vi "Lidar V3 RT Main.vi"() -> ()   [LabVIEW 2013]
uses:
  <vilib>/Platform/TimedLoop/XDataNode/timing_clust.ctl
  <vilib>/Platform/TimedLoop/XDataNode/nitl_modes.ctl
  <vilib>/Platform/TimedLoop/XDataNode/wakeup.ctl
  <vilib>/FPGAPlugInAG/PXIe-7962R/niLvFpga_Open_PXIe-7962R.vi
  <vilib>/rvi/interface/common/dynamic/niFpgaDynamicAddResources.vi
  <vilib>/FPGAPlugInAG/Dynamic/niLvFpga_Abort_Dynamic.vi
  <vilib>/FPGAPlugInAG/Dynamic/niLvFpga_Reset_Dynamic.vi
  <vilib>/FPGAPlugInAG/Dynamic/niLvFpga_Run_Dynamic.vi
  <vilib>/rvi/interface/common/niFpgaWaitOnOcc.vi
  <vilib>/Utility/error.llb/Error Cluster From Error Code.vi
  <vilib>/rvi/errors/niLvFpgaAdjustHostInterfaceError.vi
  <vilib>/FPGAPlugInAG/Dynamic/niLvFpga_Close_Dynamic.vi
  <vilib>/rvi/interface/nirviOpenFPGA/nirviOpenFPGA.xnode
  FPGA Bitfiles/LIDAR Module 5782 V3.2.lvbitx
  <vilib>/rvi/interface/nirviMethod/nirviMethod.xnode
  <vilib>/Platform/TimedLoop/XDataNode/XDataNode.xnode
  <vilib>/rvi/interface/nirviReadWriteControl/nirviReadWriteControl.xnode
  <vilib>/rvi/interface/nirviCloseFPGA/nirviCloseFPGA.xnode
  <vilib>/FPGAPlugInAG/Dynamic/niLvFpga_ReadFifo_Dynamic.vi
  <vilib>/rvi/errors/niLvFpgaMergeErrorWithErrorCode.vi
  <vilib>/ptbypt/NI_PtbyPt.lvlib
  NiFpgaLv.dll
  <vilib>/rvi/interface/Simulation/niFpgaSimulationCallBeginRW.vi
  <vilib>/Platform/TimedLoop/XDataNode/XDNodeRunTimeDep.lvlib
  <vilib>/FPGAPlugInAG/Dynamic/niLvFpga_StopFifo_Dynamic.vi
  <vilib>/FPGAPlugInAG/Dynamic/niLvFpga_ConfigureFifo_Dynamic.vi
  <vilib>/FPGAPlugInAG/Dynamic/niLvFpga_AcquireReadRegionFifo_Dynamic.vi
panel:
  out "frames counter":u32
  in  "# of Frames":u32=100
  in  "Frames Stream":bool
  in  "Frames Period":i64=100
  out "Actual Depth":u32=400384
  out "Raw Data Timeouts":u16
  in  "StreamToRawFile":bool
  in  "SingleFrame":bool
  in  "SamplingEnable":bool=TRUE
  out "Elements":i32=89152
  out "DiskWritesCounter":dbl=375.0
  out "error out 2":errorcluster
  in  "Write To File":bool
  in  "file path (use dialog)":path=path "C:/Users/LIDAR/Desktop/Scans/InterScan4.dat"
  out "error out 3":errorcluster
  out "Elements Remaining":u32
  in  "MaxStartSample":u8
  out "Intensity Map":u32[][](graph)=[[129791, 129680, 130020, 129704, 129932, 129336, 129397, 129600, 129645, 130103, 129648, 130030, 129625, 129970, 129708, 129573], [129593, 129680, 130141, 129910, 129596, 129500, 129521, 129569, 129949, 129774, 129846, 129832, 129809, 129824, 130165, 129650], [129735, 129752, 129871, 130235, 129687, 129440, 129980, 129667, 129799, 129541, 129983, 129757, 129478, 129736, 129657, 129715], [129751, 129583, 129677, 129965, 129579, 129714, 129407, 129739, 129751, 129654, 129836, 129799, 129748, 129751, 130116, 129495], [129571, 129639, 130270, 129388, 129740, 129773, 129237, 129955, 129670, 129830, 130261, 129436, 130070, 129727, 129314, 129829], [129652, 129843, 130032, 129955, 129968, 129379, 129685, 130041, 129814, 129499, 129706, 129869, 129869, 129962, 129707, 129878], [129807, 129828, 130008, 129984, 129406, 129957, 129543, 130066, 129909, 130276, 129623, 129692, 130095, 130106, 129557, 129714], [129986, 130220, 129551, 130069, 129832, 129932, 129900, 129936, 129877, 129862, 129771, 129582, 129720, 129949, 129916, 129711], [129633, 129877, 130052, 130093, 130030, 129994, 129636, 129905, 129789, 130086, 129907, 129523, 129744, 129981, 129449, 129771], [129913, 129683, 129520, 129782, 129841, 129742, 129616, 129954, 129366, 129733, 129625, 129664, 129876, 129869, 129544, 129710], [129901, 129619, 129661, 130086, 129825, 129761, 129804, 129725, 129375, 130051, 129757, 129787, 129999, 129670, 130011, 130055], [129946, 129776, 130199, 129713, 129738, 129633, 129897, 129662, 129661, 129515, 129708, 129511, 130068, 129836, 129857, 129680], [129649, 129866, 129818, 130111, 129942, 129748, 129540, 129872, 130033, 129595, 129906, 129804, 129753, 129581, 130001, 129824], [129533, 129412, 129678, 129388, 130078, 129617, 129776, 130004, 129502, 129913, 129651, 129903, 129629, 130071, 130057, 129771], [129683, 129809, 130073, 130027, 129777, 129962, 129746, 129781, 129655, 129602, 129804, 129795, 129831, 130156, 129740, 130062], [130093, 129615, 129781, 129920, 129948, 129767, 129590, 129269, 129763, 129611, 129844, 129676, 129702, 130070, 129930, 129907], [129766, 130025, 130030, 129536, 130034, 130049, 129643, 129787, 129735, 129792, 129751, 129963, 129966, 129726, 129589, 129781], [129637, 129588, 129765, 129794, 129683, 129663, 129966, 129384, 129794, 129709, 129656, 129867, 129751, 129686, 129595, 129758], [129833, 129773, 129371, 130164, 129799, 129859, 129589, 129792, 129484, 129830, 130126, 130134, 129838, 129988, 129646, 129826], [129864, 129971, 129896, 129600, 129709, 129842, 129801, 129942, 129281, 129699, 129921, 129896, 129698, 129471, 129390, 129553]]
  in  "ActiveLedIndex":u16=144
  in  "LedScanDebEn":bool
  in  "LaserPower 1":bool=TRUE
  in  "LaserPower 0":bool=TRUE
  out "Range Map":u32[][](graph)=[[63868, 63856, 63868, 63868, 63868, 63856, 63880, 63868, 63868, 63868, 63868, 63868, 63868, 63868, 63880, 63868], [63868, 63868, 63880, 63868, 63868, 63856, 63868, 63868, 63868, 63868, 63868, 63868, 63868, 63868, 63868, 63868], [63880, 63880, 63868, 63868, 63868, 63868, 63868, 63880, 63868, 63868, 63868, 63868, 63868, 63868, 63868, 63880], [63880, 63868, 63868, 63868, 63868, 63868, 63856, 63868, 63868, 63868, 63868, 63856, 63868, 63880, 63868, 63868], [63868, 63868, 63880, 63868, 63880, 63868, 63868, 63868, 63868, 63880, 63868, 63868, 63868, 63868, 63868, 63868], [63868, 63868, 63856, 63880, 63868, 63868, 63868, 63868, 63868, 63868, 63880, 63868, 63868, 63856, 63880, 63868], [63880, 63868, 63880, 63868, 63868, 63868, 63868, 63868, 63868, 63868, 63868, 63880, 63868, 63856, 63868, 63868], [63868, 63868, 63880, 63868, 63868, 63880, 63880, 63868, 63868, 63868, 63868, 63868, 63868, 63868, 63856, 63868], [63868, 63880, 63868, 63868, 63868, 63868, 63880, 63868, 63868, 63856, 63880, 63868, 63880, 63868, 63880, 63868], [63868, 63868, 63880, 63880, 63868, 63868, 63868, 63868, 63880, 63880, 63868, 63880, 63880, 63868, 63868, 63868], [63868, 63868, 63880, 63856, 63868, 63868, 63868, 63868, 63868, 63868, 63868, 63868, 63868, 63880, 63868, 63868], [63868, 63868, 63880, 63868, 63868, 63880, 63868, 63868, 63868, 63880, 63880, 63868, 63856, 63868, 63868, 63868], [63868, 63868, 63868, 63868, 63868, 63880, 63868, 63880, 63868, 63868, 63868, 63868, 63868, 63868, 63868, 63856], [63868, 63880, 63868, 63868, 63868, 63880, 63868, 63868, 63868, 63868, 63868, 63868, 63880, 63868, 63868, 63880], [63868, 63868, 63868, 63868, 63868, 63868, 63868, 63868, 63880, 63868, 63868, 63868, 63868, 63868, 63868, 63868], [63868, 63868, 63868, 63868, 63856, 63868, 63880, 63880, 63856, 63880, 63868, 63880, 63880, 63868, 63868, 63868], [63868, 63868, 63868, 63868, 63880, 63880, 63868, 63868, 63868, 63868, 63868, 63868, 63880, 63880, 63868, 63880], [63868, 63868, 63868, 63868, 63868, 63868, 63880, 63868, 63868, 63868, 63868, 63868, 63868, 63868, 63868, 63868], [63868, 63868, 63880, 63868, 63868, 63868, 63856, 63868, 63868, 63880, 63868, 63868, 63880, 63868, 63868, 63880], [63868, 63856, 63868, 63880, 63868, 63880, 63868, 63880, 63868, 63868, 63868, 63868, 63868, 63868, 63868, 63868]]
  in  "PulseEndClock":u8=4
  in  "PulseWaitClck":u16
  in  "Freq [Mhz]":dbl=125000000.0 format="%#_6p"
  out "error out":errorcluster
  out "standard deviation":dbl=5.789725206670002 format="%0.5f"
  out "Distance":dbl=63867.785252320005 format="%#.4f"
  in  "stop":bool=TRUE
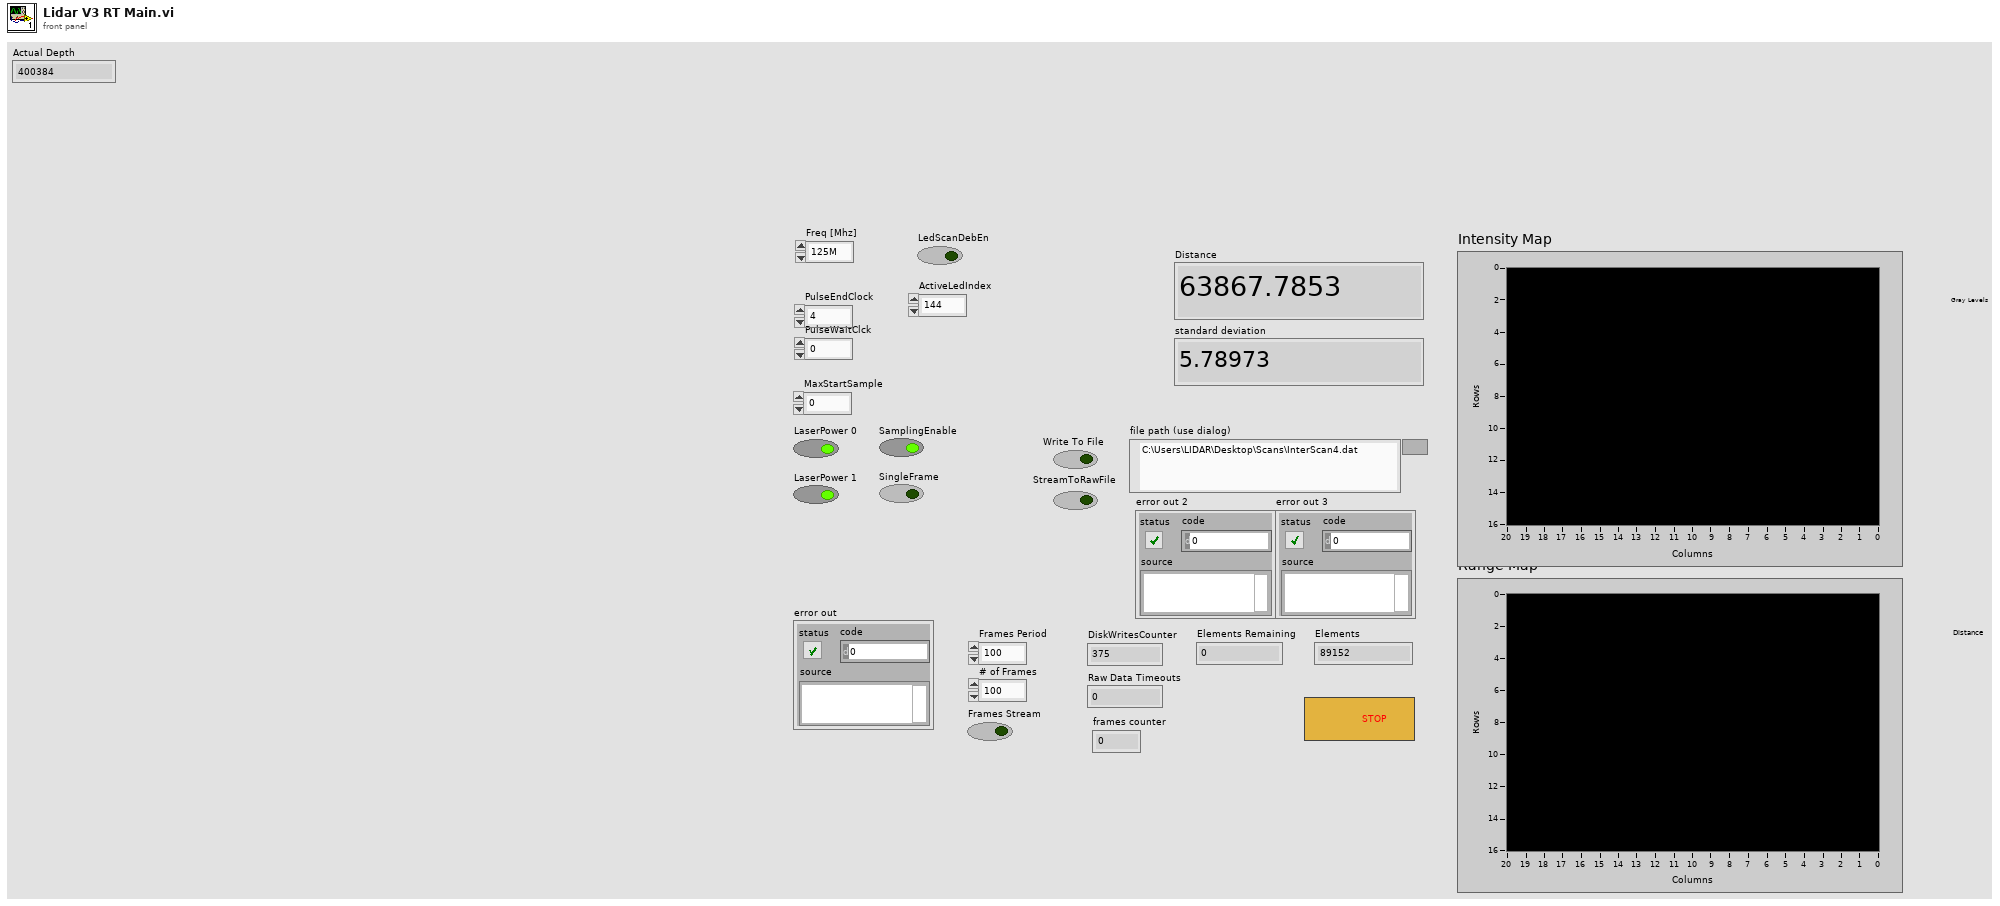
[diagram p1: front panel]
types:
  T1 = typedef "XDNodeRunTimeDep.lvlib/timing_clust.ctl" = cluster{"Expected End [f-1]":u64, "Actual End [f-1]":u64, "Finished Late? [f-1]":bool, "Expected End [i-1]":u64, "Actual End [i-1]":u64, "Finished Late? [i-1]":bool, "Expected Start [i]":u64, "Actual Start [i]":u64, "Expected Start [f]":u64, "Actual Start [f]":u64, "Source Name":string, "Structure Name":string, "Period":i64, "Deadline":i64, "Offset":i64, "Start":i64, "Priority":i32, "Timeout":i32, "Mode":T2, "Wakeup Reason":T3, "Error":errorcluster, "Source Type":string, "Secondary Source Type":string, "Global End Time":u64, "Global Start Time":u64, "Frame Duration":u64, "Iteration Duration":u64, "Assigned CPU":i32, "I/O Scan Engine Mode":u32}
  T2 = typedef "XDNodeRunTimeDep.lvlib/nitl_modes.ctl" = enum32{"No Change", "Process missed periods, maintain original phase", "Discard missed periods, maintain original phase", "Process missed periods, ignore original phase", "Discard missed periods, ignore original phase"}
  T3 = typedef "XDNodeRunTimeDep.lvlib/wakeup.ctl" = enum32{"Normal", "Aborted", "Asynchronous wakeup", "Timing source error", "Timed loop error", "Timeout"}
  T4 = enum16{"open", "replace", "create", "open or create", "replace or create", "replace or create with confirmation"}
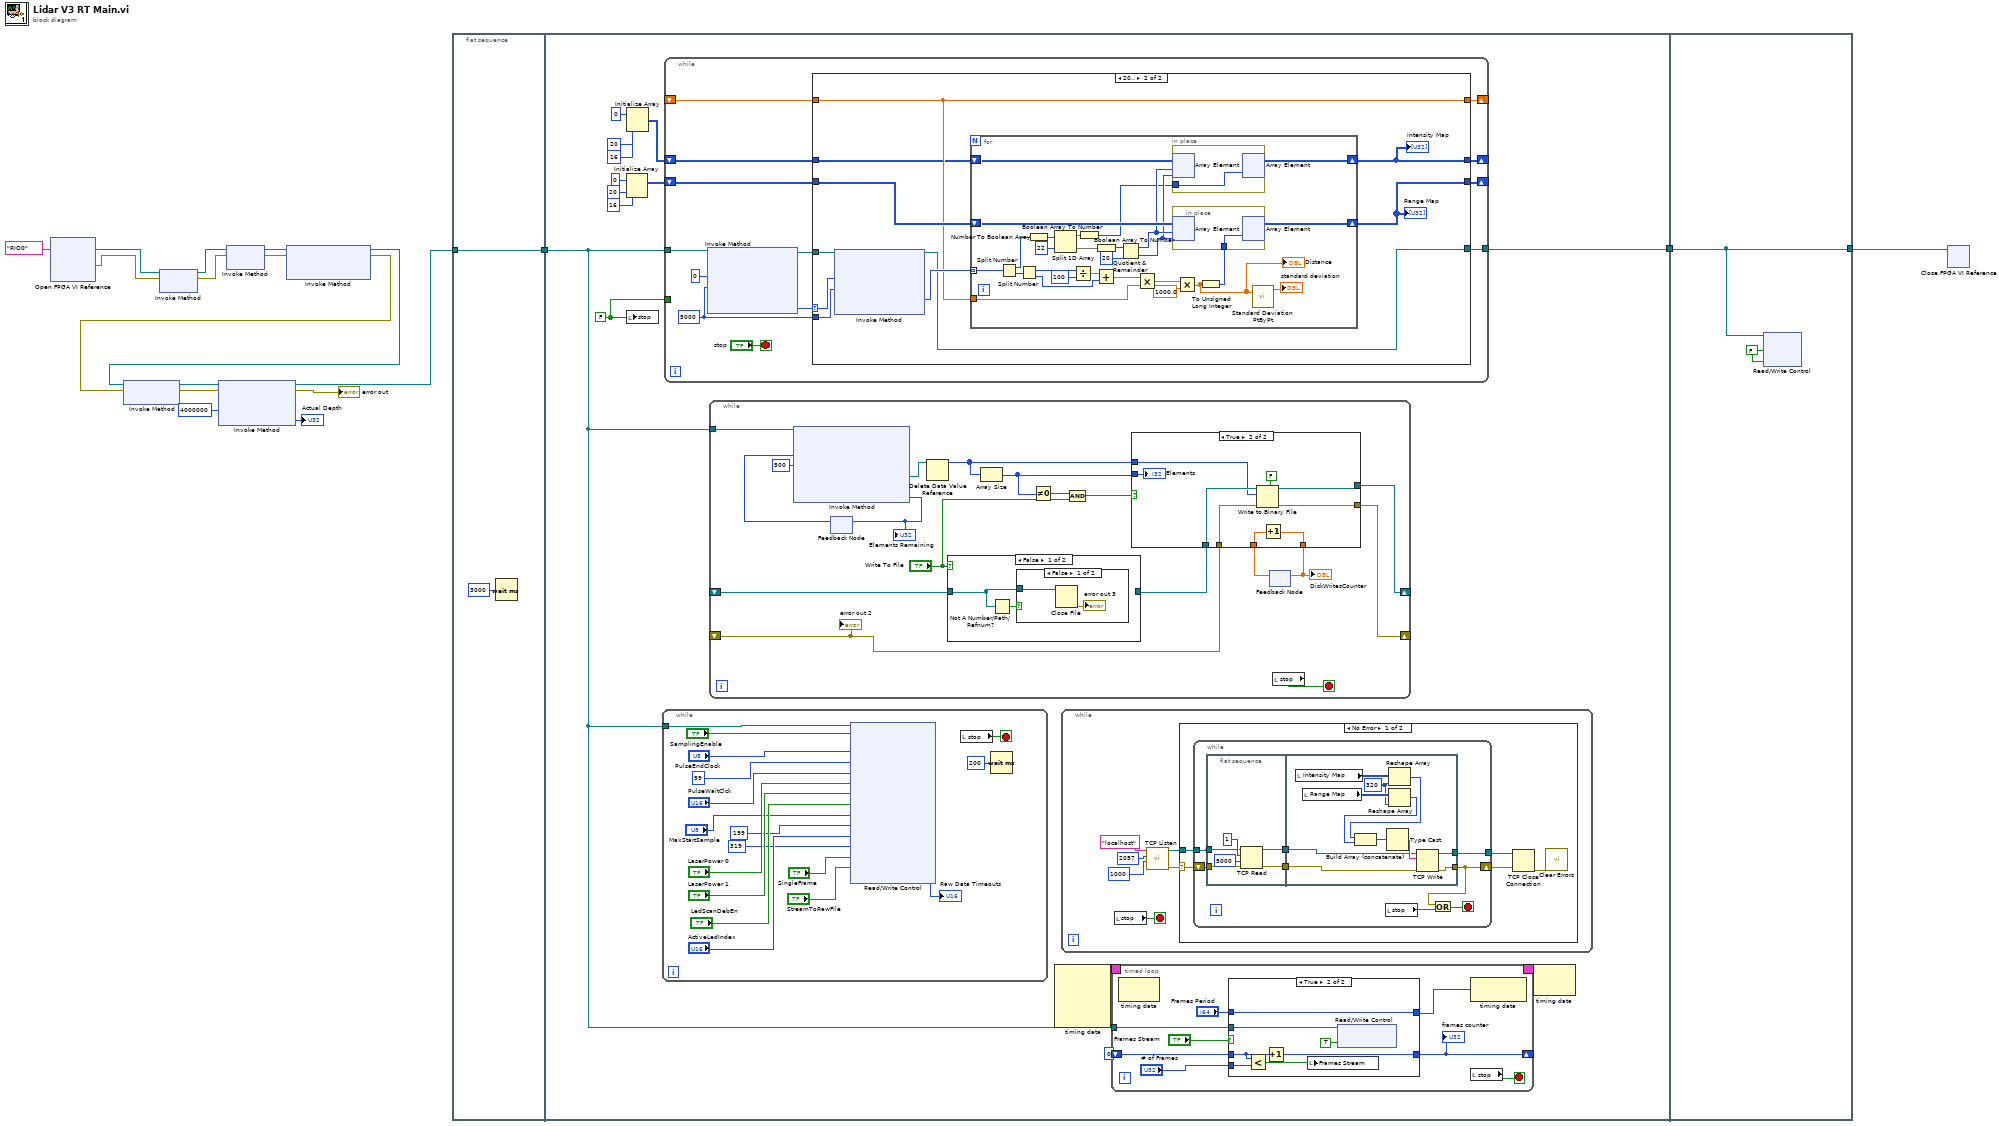
[diagram p0: block diagram]
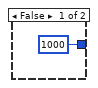
[diagram p2: hidden frame]
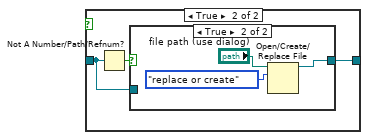
[diagram p4: hidden frame]
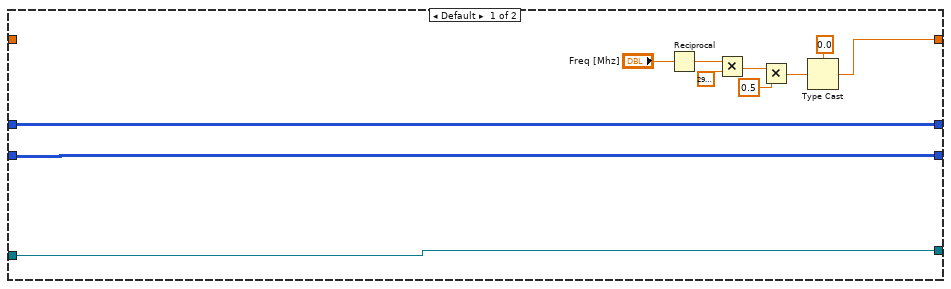
[diagram p8: hidden frame]
diagram:
  n1 = xnode "Open FPGA VI Reference"("resource name"=tag "RIO0") -> ("FPGA VI Reference Out"=w12:refnum<k20>, "error out"=w10:errorcluster)  [unwired: 1 in]
  n2 = xnode "Invoke Method"("FPGA VI Reference In"=w12, "error in"=w10) -> ("FPGA VI Reference Out"=w11:refnum<k20>, "error out"=w9:errorcluster)
  n3 = xnode "Invoke Method"("FPGA VI Reference In"=w11, "error in"=w9) -> ("FPGA VI Reference Out"=w16:refnum<k20>, "error out"=w15:errorcluster)
  n4 = xnode "Invoke Method"("FPGA VI Reference In"=w16, "error in"=w15) -> ("FPGA VI Reference Out"=w2:refnum<k20>, "error out"=w4:errorcluster)  [unwired: 1 in]
  n5 = xnode "Invoke Method"("FPGA VI Reference In"=w2, "error in"=w4) -> ("FPGA VI Reference Out"=w7:refnum<k20>, "error out"=w8:errorcluster)
  n6 = xnode "Invoke Method"("FPGA VI Reference In"=w7, "error in"=w8, "Requested Depth"=u32 4000000) -> ("FPGA VI Reference Out"=w1:refnum<k20>, "error out"=→"error out":errorcluster, "Actual Depth"=→"Actual Depth":u32)
  n7 = flat-sequence {
    tunnel: w1 -> [w20]
    tunnel: [w20] -> w14
    tunnel: w14 -> [w22]
    tunnel: [w34] -> w13
    tunnel: [w215] -> w17
    tunnel: w13 -> [w215]
    frame #0 {
      n8 = Wait (ms)(milliseconds to wait=u32 3000) -> ()  [unwired: 1 out]
    }
    frame #1 {
      w33 = FALSE ("stop")
      n9 = Initialize Array(u32 0 ("element"), 20 ("dimension size"), 16 ("dimension size")) -> (w29:u32[][])
      n10 = local write "stop"(w33) -> ()
      n11 = Initialize Array(u32 0 ("element"), 20 ("dimension size"), 16 ("dimension size")) -> (w25:u32[][])
      n12 = while {
        tunnel: w22 -> [w147]
        stop <- w146 stop-if-true
        n13 = xnode "Read/Write Control"("FPGA VI Reference In"=w147, "SamplingEnable"="SamplingEnable", "PulseEndClck"="PulseEndClock", "SampPerPulse"=u8 99, "PulseWaitClck"="PulseWaitClck", "PFI2"="LaserPower 0", "PFI3"="LaserPower 1", "LedScanDebEn"="LedScanDebEn", "MaxStartSample"="MaxStartSample", "PulsePerLed"=i16 199, "ActiveLedIndexDeb"="ActiveLedIndex", "NoOfLeds"=u16 319, "SingleFrame"="SingleFrame", "StreamToDMA"="StreamToRawFile") -> ("Timeouts"=→"Raw Data Timeouts":u16)  [unwired: 1 in, 2 out]
        n14 = local read "stop"() -> (w146:bool)
        n15 = Wait (ms)(milliseconds to wait=u32 200) -> ()  [unwired: 1 out]
      }
      n16 = while {
        tunnel: w22 -> [w163]
        tunnel: [w158] -> w34
        tunnel: w33 -> [_]
        shift-right: [w156] -> _
        shift-left: _ -> [w155]
        shift-right: [w153] -> _
        shift-left: w29 -> [w154]
        shift-right: [w151] -> _
        shift-left: w25 -> [w152]
        stop <- "stop" stop-if-true
        w160 = 5000 ("Timeout (ms)")
        n17 = xnode "Invoke Method"("FPGA VI Reference In"=w163, "Number of Elements"=u32 0, "Timeout (ms)"=w160) -> ("FPGA VI Reference Out"=w161:refnum<k20>, "Elements Remaining"=w157:u32)  [unwired: 1 in, 2 out]
        n18 = case shown="20.." w157 {
          selector: w157 -> [_ w175]
          tunnel: w161 -> [w174 w184]
          tunnel: w160 -> [_ w183]
          tunnel: [w174 w181] -> w158
          tunnel: [w166 w179] -> w156
          tunnel: w155 -> [_ w179]
          tunnel: w154 -> [w165 w180]
          tunnel: [w165 w178] -> w153
          tunnel: w152 -> [w164 w177]
          tunnel: [w164 w176] -> w151
          frame Default {
            n19 = Reciprocal(x="Freq [Mhz]") -> (1/x=w173:dbl)
            n20 = Multiply(x=w173, y=dbl[unit] 299792458.0) -> (x*y=w170:dbl[unit])
            n21 = Multiply(x=w170, y=dbl[unit] 0.5) -> (x*y=w167:dbl[unit])
            n22 = Type Cast(type=0.0 ("y"), x=w167) -> (*(type *) &x=w166:dbl)
          }
          frame 20.. {
            n23 = xnode "Invoke Method"("FPGA VI Reference In"=w184, "Number of Elements"=w175, "Timeout (ms)"=w183) -> ("FPGA VI Reference Out"=w181:refnum<k20>, "Data"=w182:u64[])  [unwired: 1 in, 2 out]
            n24 = for {
              tunnel: w182 -> [w211] mode=indexing
              shift-right: [w207] -> w178
              shift-left: w180 -> [w208]
              tunnel: w179 -> [w206]
              shift-right: [w202] -> w176
              shift-left: w177 -> [w203]
              n25 = Split Number(x=w211) -> (hi(x)=w209:u32, lo(x)=w210:u32)
              n26 = Split Number(x=w210) -> (hi(x)=w204:u16, lo(x)=w201:u16)
              n27 = Number To Boolean Array(number=w209) -> (Boolean array=w200:bool[])
              n28 = Split 1D Array(array=w200, index=22) -> (first subarray=w187:bool[], second subarray=w198:bool[])
              n29 = Divide(x=w204, y=u16 100) -> (x/y=w194:dbl)
              n30 = Boolean Array To Number(Boolean array=w187) -> (number=w186:u32)
              n31 = Add(x=w194, y=w201) -> (x+y=w195:dbl)
              n32 = Boolean Array To Number(Boolean array=w198) -> (number=w197:u32)
              n33 = Quotient & Remainder(x=w197, y=u32 20) -> (x-y*floor(x/y)=w189:u32, floor(x/y)=w188:u32)
              n34 = Multiply(x=w195, y=w206) -> (x*y=w191:dbl)
              n35 = in-place {
                in-place-border: w186 -> [w212]
                n36 = in-place-array #1(w203, w189, w188) -> ()  [unwired: 1 out]
                n37 = in-place-array #1(w212) -> (w202:u32[][])  [unwired: 2 out]
              }
              n38 = Multiply(x=w191, y=1000.0) -> (x*y=w185:dbl)
              "Distance" <- w185
              n39 = To Unsigned Long Integer(number=w185) -> (unsigned 32bit integer=w205:u32)
              n40 = in-place {
                in-place-border: w205 -> [w213]
                n41 = in-place-array #2(w208, w189, w188) -> ()  [unwired: 1 out]
                n42 = in-place-array #2(w213) -> (w207:u32[][])  [unwired: 2 out]
              }
              n43 = call <vilib>:"Standard Deviation PtByPt.vi"("x"=w185) -> ("standard deviation"=→"standard deviation":dbl)  [unwired: 2 in, 2 out]
            }
            "Range Map" <- w178
            "Intensity Map" <- w176
          }
        }
      }
      n44 = while {
        tunnel: w22 -> [w74]
        shift-right: [w73] -> _
        shift-left: _ -> [w66]
        shift-right: [w72] -> _
        shift-left: _ -> [w71]
        stop <- w57 stop-if-true
        n45 = feedback #3() -> (w58:u32)  [unwired: 1 in]
        n46 = xnode "Invoke Method"("FPGA VI Reference In"=w74, "Number of Elements"=w58, "Timeout (ms)"=500) -> ("Read Region Reference"=w68:refnum<data-value>, "Elements Remaining"=w59:u32)  [unwired: 1 in, 3 out]
        "Elements Remaining" <- w59
        n47 = feedback-in #3(w59) -> ()
        n48 = Delete Data Value Reference(data value reference=w68) -> (data value=w62:u32[])  [unwired: 1 in, 1 out]
        n49 = case shown="False" "Write To File" {
          tunnel: w66 -> [w75 w79]
          tunnel: [_ w81] -> w65
          frame False {
            n50 = Not A Number/Path/Refnum?(number/path/refnum=w75) -> (NaN/Path/Refnum?=w76:bool)
            n51 = case shown="False" w76 {
              tunnel: w75 -> [w78 _]
              frame False {
                n52 = Close File(refnum=w78) -> (error out=→"error out 3":errorcluster)  [unwired: 1 in, 1 out]
              }
              frame True {
              }
            }
          }
          frame True {
            n53 = Not A Number/Path/Refnum?(number/path/refnum=w79) -> (NaN/Path/Refnum?=w80:bool)
            n54 = case shown="True" w80 {
              tunnel: [w82 w83] -> w81
              tunnel: w79 -> [w82 _]
              frame False {
              }
              frame True {
                n55 = Open/Create/Replace File(file path (use dialog)="file path (use dialog)", operation (0:open)=T4."replace or create") -> (refnum out=w83:refnum<file>)  [unwired: 4 in, 2 out]
              }
            }
          }
        }
        n56 = Array Size(array=w62) -> (size(s)=w61:i32)
        n57 = Not Equal To 0?(x=w61) -> (x != 0?=w60:bool)
        n58 = And(x=w60, y="Write To File") -> (x .and. y?=w67:bool)
        n59 = feedback #4() -> (w69:dbl)  [unwired: 1 in]
        n60 = case shown="True" w67 {
          tunnel: [w86 w96] -> w73
          tunnel: w71 -> [w88 w91]
          tunnel: [w88 w95] -> w72
          tunnel: [w87 w93] -> w70
          tunnel: w69 -> [w87 w94]
          tunnel: w62 -> [_ w90]
          tunnel: w65 -> [w86 w92]
          tunnel: w61 -> [_ w89]
          frame False {
          }
          frame True {
            n61 = Write to Binary File(file (use dialog)=w92, data=w90, error in=w91, 5:FALSE ("prepend array or string size? (T)")) -> (refnum out=w96:refnum<file>, error out=w95:errorcluster)  [unwired: 2 in, 1 out]
            n62 = Increment(x=w94) -> (x+1=w93:dbl)
            "Elements" <- w89
          }
        }
        "DiskWritesCounter" <- w70
        n63 = feedback-in #4(w70) -> ()
        n64 = local read "stop"() -> (w57:bool)
        "error out 2" <- w71
      }
      n65 = node-c288() -> (w24:T1)  [unwired: 4 in]
      n66 = while {
        stop <- w99 stop-if-true
        n67 = local read "stop"() -> (w99:bool)
        n68 = call <vilib>:"TCP Listen.vi"("timeout ms (wait forever: -1)"=1000, "port"=u16 2057, "service name"="localhost" ("address")) -> ("error out"=w98:errorcluster, "connection ID"=w103:refnum<k5>)  [unwired: 4 in, 3 out]
        n69 = case shown="No Error" w98 {
          selector: w98 -> [w104 _]
          tunnel: w103 -> [w106 _]
          frame No Error {
            n70 = while {
              tunnel: w106 -> [w116]
              tunnel: [w111] -> w107
              shift-right: [w109] -> w108
              shift-left: w104 -> [w115]
              stop <- w110 stop-if-true
              n71 = flat-sequence {
                tunnel: w116 -> [w119]
                tunnel: w115 -> [w118]
                tunnel: [w122] -> w113
                tunnel: [w121] -> w112
                tunnel: w113 -> [w131]
                tunnel: w112 -> [w130]
                tunnel: [w129] -> w111
                tunnel: [w128] -> w109
                frame #0 {
                  n72 = TCP Read(connection ID=w119, bytes to read=1, error in (no error)=w118, 9:5000 ("timeout ms (25000)")) -> (connection ID out=w122:refnum<k5>, error out=w121:errorcluster)  [unwired: 1 in, 1 out]
                }
                frame #1 {
                  w123 = 320 ("dimension size")
                  n73 = local read "Intensity Map"() -> (w127:u32[][])
                  n74 = local read "Range Map"() -> (w133:u32[][])
                  n75 = Reshape Array(w127, w123) -> (w126:u32[])
                  n76 = Reshape Array(w133, w123) -> (w125:u32[])
                  n77 = Build Array (concatenate)(w126, w125) -> (w124:u32[])
                  n78 = Type Cast(x=w124) -> (*(type *) &x=w132:string)  [unwired: 1 in]
                  n79 = TCP Write(connection ID=w131, data in=w132, error in (no error)=w130) -> (connection ID out=w129:refnum<k5>, error out=w128:errorcluster)  [unwired: 1 in, 1 out]
                }
              }
              n80 = local read "stop"() -> (w114:bool)
              n81 = Or(x=w109, y=w114) -> (x .or. y?=w110:bool)
            }
            n82 = TCP Close Connection(connection ID=w107, error in (no error)=w108) -> (error out=w105:errorcluster)  [unwired: 1 in, 1 out]
            n83 = call <vilib>:"Clear Errors.vi"("error in (no error)"=w105) -> ()  [unwired: 6 in, 1 out]
          }
          frame Error {
          }
        }
      }
      n84 = timed-loop {
        timing: w24 -> [_]
        timing-out: [_] -> w23
        tunnel: w22 -> [w42]
        shift-right: [w35] -> _
        shift-left: u32 0 ("# of Frames") -> [w38]
        stop <- w39 stop-if-true
        n85 = node-c288() -> ()  [unwired: 1 in, 1 out]
        n86 = case shown="True" "Frames Stream" {
          tunnel: w42 -> [_ w49]
          tunnel: [i64 1000 ("Frames Period") w48] -> w40
          tunnel: "Frames Period" -> [_ w48]
          tunnel: w38 -> [_ w46]
          tunnel: [_ w47] -> w35
          tunnel: "# of Frames" -> [_ w45]
          frame False {
          }
          frame True {
            n87 = Less?(x=w46, y=w45) -> (x < y?=w44:bool)
            n88 = Increment(x=w46) -> (x+1=w47:u32)
            n89 = local write "Frames Stream"(w44) -> ()
            n90 = xnode "Read/Write Control"("FPGA VI Reference In"=w49, "SingleFrame"=TRUE) -> ()  [unwired: 1 in, 2 out]
          }
        }
        "frames counter" <- w35
        n91 = node-c288(w40) -> ()  [unwired: 1 out]
        n92 = local read "stop"() -> (w39:bool)
      }
      n93 = node-c288(w23) -> ()  [unwired: 1 out]
    }
    frame #2 {
      w214 = FALSE ("PFI2")
      n94 = xnode "Read/Write Control"("FPGA VI Reference In"=w215, "PFI2"=w214, "PFI3"=w214) -> ()  [unwired: 1 in, 2 out]
    }
  }
  n95 = xnode "Close FPGA VI Reference"("FPGA VI Reference In"=w17) -> ()  [unwired: 1 in, 1 out]
